vi "XY Graph Save Plot Event.vi"(6 "Delimiter (TAB)":string="\t", 8 "Error In":errorcluster, 9 "Mouse Click Coordinates":T1, 11 "XYGraph Ref":T2) -> (0 "Error Out":errorcluster, 1 "Message":string, 2 "File Path":path, 3 "Plot Name":string, 4 "Saved Plot Index":i32, 5 "Graph Caption":string)   [LabVIEW 2019, in "XY Graph Add-Ons.lvlib"]
uses:
  XY Graph Add-Ons.lvlib
  XY Graph Refnum.ctl
  <vilib>/Utility/miscctls.llb/LVPoint32TypeDef.ctl
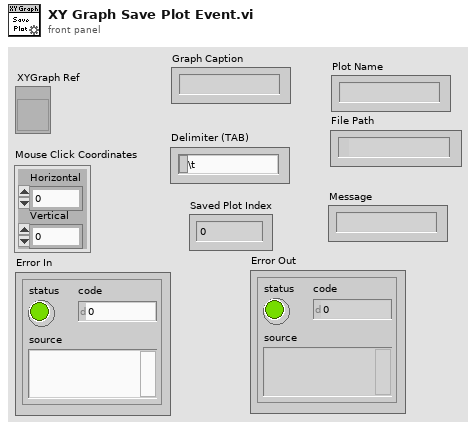
[diagram p1: front panel]
types:
  T1 = typedef "LVPoint32TypeDef.ctl" = cluster{"Horizontal":i32, "Vertical":i32}
  T2 = typedef "XY Graph Add-Ons.lvlib/XY Graph Refnum.ctl" = refnum<vi>
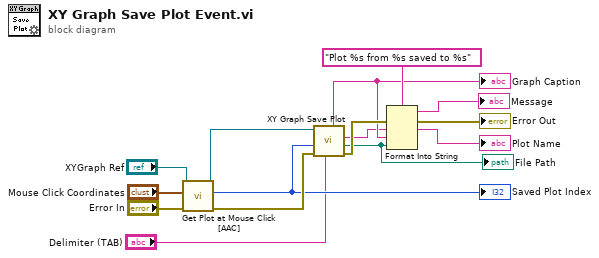
[diagram p0: block diagram]
diagram:
  n1 = call "Get Plot at Mouse Click [AAC].vi"("error in (no error)"="Error In", "Mouse Click Coordinates"="Mouse Click Coordinates", "XYGraph Ref"="XYGraph Ref") -> ("error out"=w10:errorcluster, "Plot at Coordinates"=w9:i32, "XYGraph Ref"=w12:T2)  [unwired: 2 in, 4 out]
  "Saved Plot Index" <- w9
  n2 = call "XY Graph Save Plot.vi"("Delimiter (TAB)"="Delimiter (TAB)", "Error In"=w10, "Plot Index"=w9, "XYGraph Ref"=w12) -> ("Error Out"=w6:errorcluster, "File Path"=w5:path, "Plot Name"=w1:string, "Graph Caption"=w2:string)  [unwired: 3 in, 1 out]
  "Graph Caption" <- w2
  "Plot Name" <- w1
  "File Path" <- w5
  n3 = Format Into String(format string="Plot %s from %s saved to %s", error in=w6, w1, w2, w5) -> (resulting string=→"Message":string, error out=→"Error Out":errorcluster)  [unwired: 1 in]
